vi "小时数据发送 (子VI).vi"(11 "数值":i32) -> (0 "error out":errorcluster)   [LabVIEW 2016, in "数据传输系统.lvlib"]
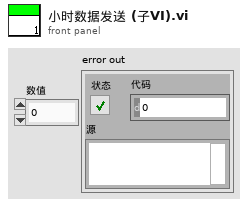
[diagram p1: front panel]
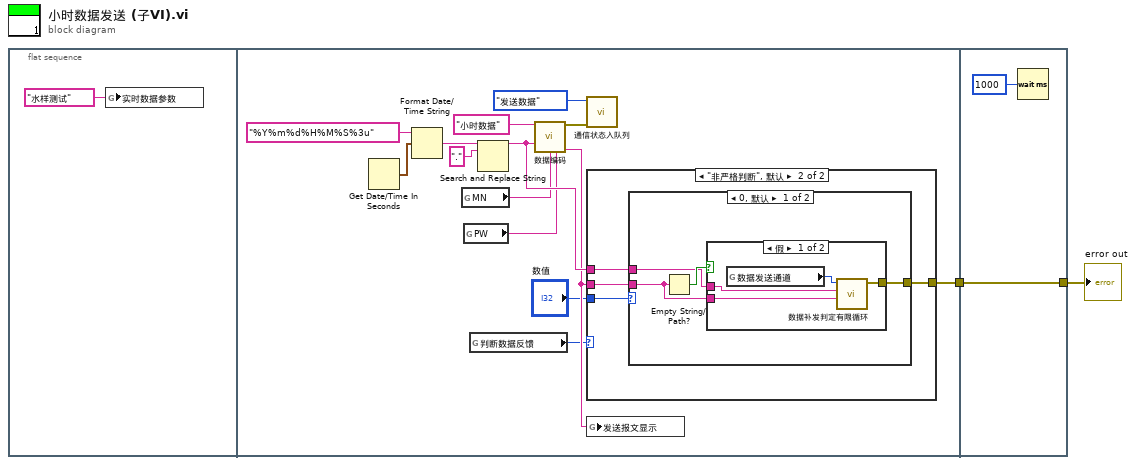
[diagram p0: block diagram]
diagram:
  n1 = flat-sequence {
    tunnel: [w4] -> w1
    tunnel: [w31] -> w2
    tunnel: w1 -> [w31]
    frame #0 {
      n2 = global write "全局 实时数据参数.vi" "实时数据参数"("水样测试" ("实时数据参数")) -> ()
    }
    frame #1 {
      n3 = Get Date/Time In Seconds() -> (seconds since 1Jan1904=w8:timestamp)
      n4 = Format Date/Time String(time format string (%c)="%Y%m%d%H%M%S%3u" ("时间格式字符串(%c)"), seconds (now)=w8) -> (date/time string=w7:string)  [unwired: 1 in]
      n5 = global read "断电保存全局.vi" "MN"() -> (w11:string)
      n6 = global read "断电保存全局.vi" "PW"() -> (w12:string)
      n7 = global read "断电保存全局.vi" "判断数据反馈"() -> (w15:enum16{"非严格判断", "严格判断", "不判断"})
      n8 = Search and Replace String(input string=w7, search string="." ("搜索字符串")) -> (result string=w17:string)  [unwired: 6 in, 3 out]
      n9 = call "数据编码.vi"("table输入"="小时数据" ("新元素/子数组"), "QN"=w17, "MN"=w11, "PW"=w12) -> ("错误常量"=w14:errorcluster, "通讯包字符串"=w16:string)  [unwired: 10 in]
      n10 = call "通信状态入队列.vi"("错误输入（无错误）"=w14, "枚举"=enum16{"打开连接", "发送数据", "读取数据", "数据处理", "关闭连接"}."发送数据") -> ()  [unwired: 9 in, 1 out]
      n11 = case shown="\"非严格判断\", 默认" w15 {
        tunnel: [_ w21] -> w4
        tunnel: w16 -> [_ w20]
        tunnel: "数值" -> [_ w19]
        tunnel: w17 -> [_ w18]
        frame "不判断" {
        }
        frame "非严格判断", Default {
          n12 = case shown="0, 默认" w19 {
            tunnel: [w24 _] -> w21
            tunnel: w20 -> [w23 _]
            tunnel: w18 -> [w22 _]
            frame 0, Default {
              n13 = Empty String/Path?(string/path=w23) -> (empty?=w25:bool)
              n14 = case shown="假" w25 {
                tunnel: [w29 _] -> w24
                tunnel: w23 -> [w28 _]
                tunnel: w22 -> [w26 _]
                frame False {
                  n15 = global read "断电保存全局.vi" "数据发送通道"() -> (w27:enum16{"TCP", "VISA"})
                  n16 = call "数据补发判定有限循环.vi"("数据输入"=w28, "QN"=w26, "数据发送通道"=w27) -> ("error out"=w29:errorcluster)  [unwired: 8 in]
                }
                frame True {
                }
              }
            }
            frame 14..17, 27..30 {
              # "流量数据"
            }
          }
        }
      }
      n17 = global write "全局1.vi" "发送报文显示"(w16) -> ()
    }
    frame #2 {
      n18 = Wait (ms)(milliseconds to wait=u32 1000 ("等待时间（毫秒）")) -> ()  [unwired: 1 out]
    }
  }
  "error out" <- w2
